vi "Pick from Available Cells.vi"(0 "Available Cells":bool[][](array[boolean]), 11 "error in (no error)":errorcluster) -> (4 "Picked Cell #":i32, 10 "Free Cell?":bool, 15 "error out":errorcluster)   [LabVIEW 2014, in "Dragon Tamers.lvlib"]
uses:
  Dragon Tamers.lvlib
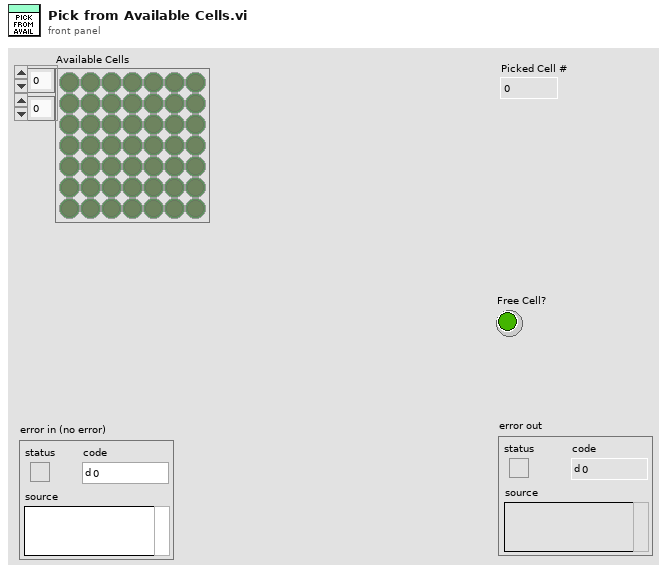
[diagram p1: front panel]
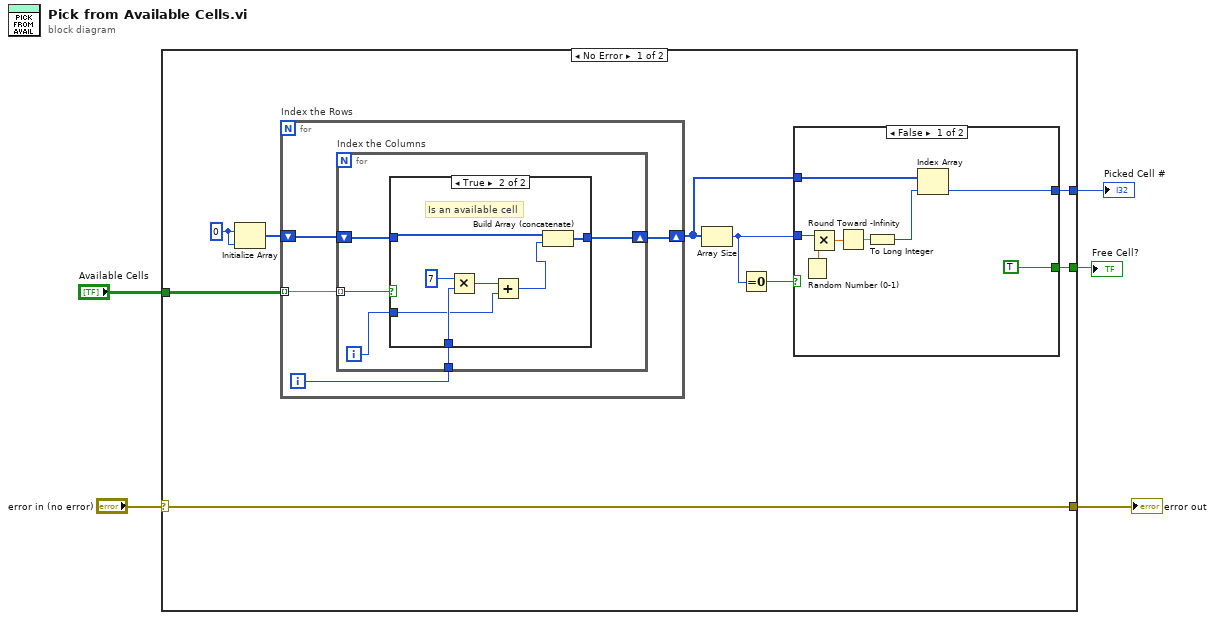
[diagram p0: block diagram]
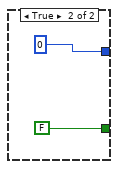
[diagram p2: hidden frame]
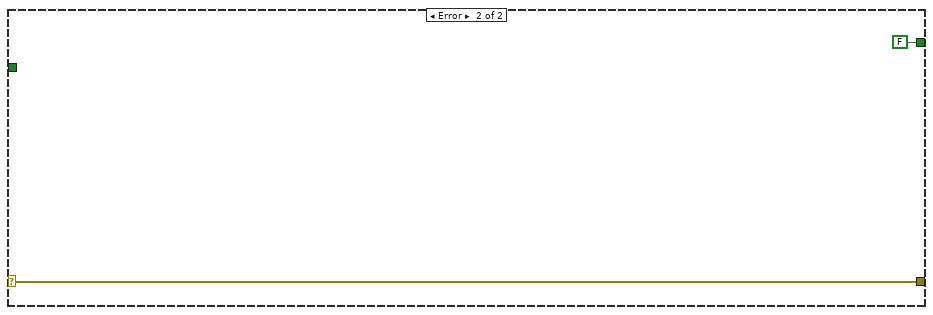
[diagram p4: hidden frame]
diagram:
  n1 = case shown="No Error" "error in (no error)" {
    selector: "error in (no error)" -> [w14 w43]
    tunnel: [w14 w43] -> w4
    tunnel: "Available Cells" -> [w13 _]
    tunnel: [w8 _] -> w2
    tunnel: [w6 FALSE] -> w1
    frame No Error {
      w11 = 0
      n2 = Initialize Array(w11, w11) -> (w12:i32[])
      n3 = for "Index the Rows" {
        tunnel: w13 -> [w28] mode=indexing
        shift-right: [w25] -> w7
        shift-left: w12 -> [w27]
        i -> [w26]
        n4 = for "Index the Columns" {
          tunnel: w28 -> [w33] mode=indexing
          shift-right: [w29] -> w25
          shift-left: w27 -> [w32]
          tunnel: w26 -> [w31]
          i -> [w30]
          n5 = case shown="True" w33 {
            tunnel: w32 -> [w34 w36]
            tunnel: w31 -> [_ w41]
            tunnel: w30 -> [_ w38]
            tunnel: [w34 w35] -> w29
            frame False {
            }
            frame True {
              # "Is an available cell"
              n6 = Multiply(x=7, y=w41) -> (x*y=w39:i32)
              n7 = Add(x=w39, y=w38) -> (x+y=w37:i32)
              n8 = Build Array (concatenate)(w36, w37) -> (w35:i32[])
            }
          }
        }
      }
      n9 = Array Size(array=w7) -> (size(s)=w10:i32)
      n10 = Equal To 0?(x=w10) -> (x = 0?=w9:bool)
      n11 = case shown="False" w9 {
        tunnel: w10 -> [w22 _]
        tunnel: [w18 0] -> w8
        tunnel: w7 -> [w19 _]
        tunnel: [TRUE FALSE] -> w6
        frame False {
          n12 = Random Number (0-1)() -> (number: 0 to 1=w21:dbl)
          n13 = Multiply(x=w22, y=w21) -> (x*y=w20:dbl)
          n14 = Round Toward -Infinity(1:w20) -> (0:w17:dbl)
          n15 = To Long Integer(number=w17) -> (32bit integer=w16:i32)
          n16 = Index Array(array=w19, index=w16) -> (element=w18:i32)
        }
        frame True {
        }
      }
    }
    frame Error {
    }
  }
  "error out" <- w4
  "Picked Cell #" <- w2
  "Free Cell?" <- w1
